vi "LWXPS_ControllerSlaveStatusGet.vi"(0 "XPS Reference IN":refnum<k24>, 11 "LabVIEW error IN":errorcluster caption="error in") -> (4 "XPS Reference OUT":refnum<k24>, 6 "Returned error code":i32, 8 "Slave Controller Status":i32, 10 "XPS Error String":string, 15 "LabVIEW error OUT":errorcluster)   [LabVIEW 2014]
uses:
  D:/XPSQ8_LabView_Library/Development/Source/Dll/Newport.XPS.CommandInterface.dll
  Dll/Newport.XPS.CommandInterface.dll
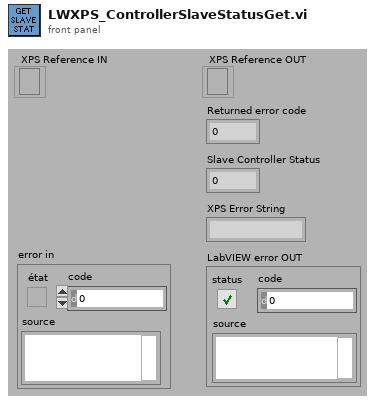
[diagram p1: front panel]
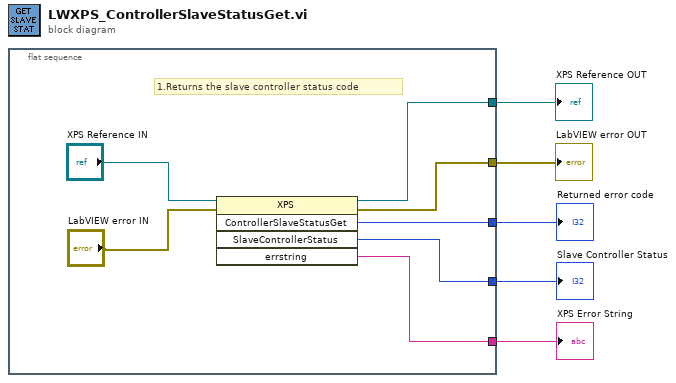
[diagram p0: block diagram]
diagram:
  n1 = flat-sequence {
    tunnel: [w6] -> w5
    tunnel: [w12] -> w4
    tunnel: [w11] -> w2
    tunnel: [w8] -> w3
    tunnel: [w7] -> w1
    frame #0 {
      # "1.Returns the slave controller status code"
      n2 = invoke class="XPS" method="ControllerSlaveStatusGet"(reference="XPS Reference IN", error in="LabVIEW error IN") -> (reference out=w6:refnum<k24>, error out=w12:errorcluster, "ControllerSlaveStatusGet"=w8:i32, "SlaveControllerStatus"=w11:i32, "errstring"=w7:string)  [unwired: 3 in]
    }
  }
  "XPS Reference OUT" <- w5
  "LabVIEW error OUT" <- w4
  "Returned error code" <- w3
  "Slave Controller Status" <- w2
  "XPS Error String" <- w1
